vi "Teleop.vi"(10 "Match Info":T1={"Autonomous Elapsed Seconds"=0.0, "TeleOp Elapsed Seconds"=0.0, "Disabled Elapsed Seconds"=0.0, "Visited Autonomous"=FALSE, "Visited TeleOp"=FALSE, "Visited Disabled"=FALSE, "Autonomous Settings"={"Autonomous Style"=enum."Independent", "VI Refnum"=refnum}}, 11 "Call Context":T2) -> ()   [LabVIEW 2017]
doc: "This VI is called for each TeleOp packet received from the DS where the robot is not disabled. It is often used to read from the joysticks and update I/O or to update setpoints for timed control loops. It should complete and return within 20 milliseconds or it may miss DS packets."
uses:
  <vilib>/Rock Robotics/WPI/DriverStation/WPI_DriverStationDerivedRobotMode.ctl
  <vilib>/Rock Robotics/WPI/DriverStation/WPI_DriverStationMatch Info.ctl
  <vilib>/Rock Robotics/WPI/Utilities/WPI_GetSetVariantRefNum.vi
  <vilib>/Rock Robotics/Network Tables/NT Write Boolean Array.vi
  <vilib>/Rock Robotics/Network Tables/NT Write Numeric Array.vi
  <vilib>/Rock Robotics/Network Tables/NT Read Boolean.vi
  <vilib>/Rock Robotics/Network Tables/NT Read Number.vi
  Robot Global Data.vi
panel:
  out "Sample Slider 0":dbl(slide) scale=0.0..5.0
  out "Sample Boolean 1":bool
  out "Sample Boolean 0":bool
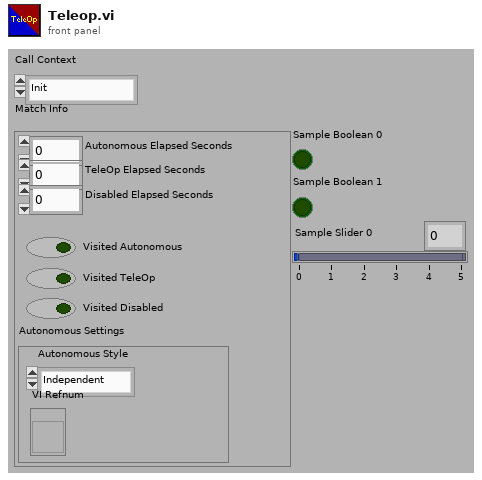
[diagram p1: front panel]
types:
  T1 = typedef "WPI_DriverStationMatch Info.ctl" = cluster{"Autonomous Elapsed Seconds":dbl, "TeleOp Elapsed Seconds":dbl, "Disabled Elapsed Seconds":dbl, "Visited Autonomous":bool, "Visited TeleOp":bool, "Visited Disabled":bool, "Autonomous Settings":cluster{"Autonomous Style":enum16{"Iterative", "Independent"}, "VI Refnum":refnum<vi>}}
  T2 = typedef "WPI_DriverStationDerivedRobotMode.ctl" = enum16{"Init", "Execute", "Stop"}
  T3 = typedef "WPI_JoystickDevRef.ctl" = cluster{"Device":T4}
  T4 = typedef "WPI_JoystickDeviceEnum.ctl" = enum16{"USB 0", "USB 1", "USB 2", "USB 3", "USB 4", "USB 5"}
  T5 = enum16{"SingleJoystick", "DoubleJoystick", "GameController"}
  T6 = cluster{"Buttons[0]":bool, "Buttons[1]":bool, "Buttons[2]":bool, "Buttons[3]":bool, "Buttons[4]":bool, "Buttons[5]":bool, "Buttons[6]":bool, "Buttons[7]":bool, "Buttons[8]":bool}
  T7 = cluster{"Axes[0]":dbl, "Axes[1]":dbl, "Axes[2]":dbl, "Axes[3]":dbl, "Axes[4]":dbl, "Axes[5]":dbl, "Axes[6]":dbl, "Axes[7]":dbl, "Axes[8]":dbl}
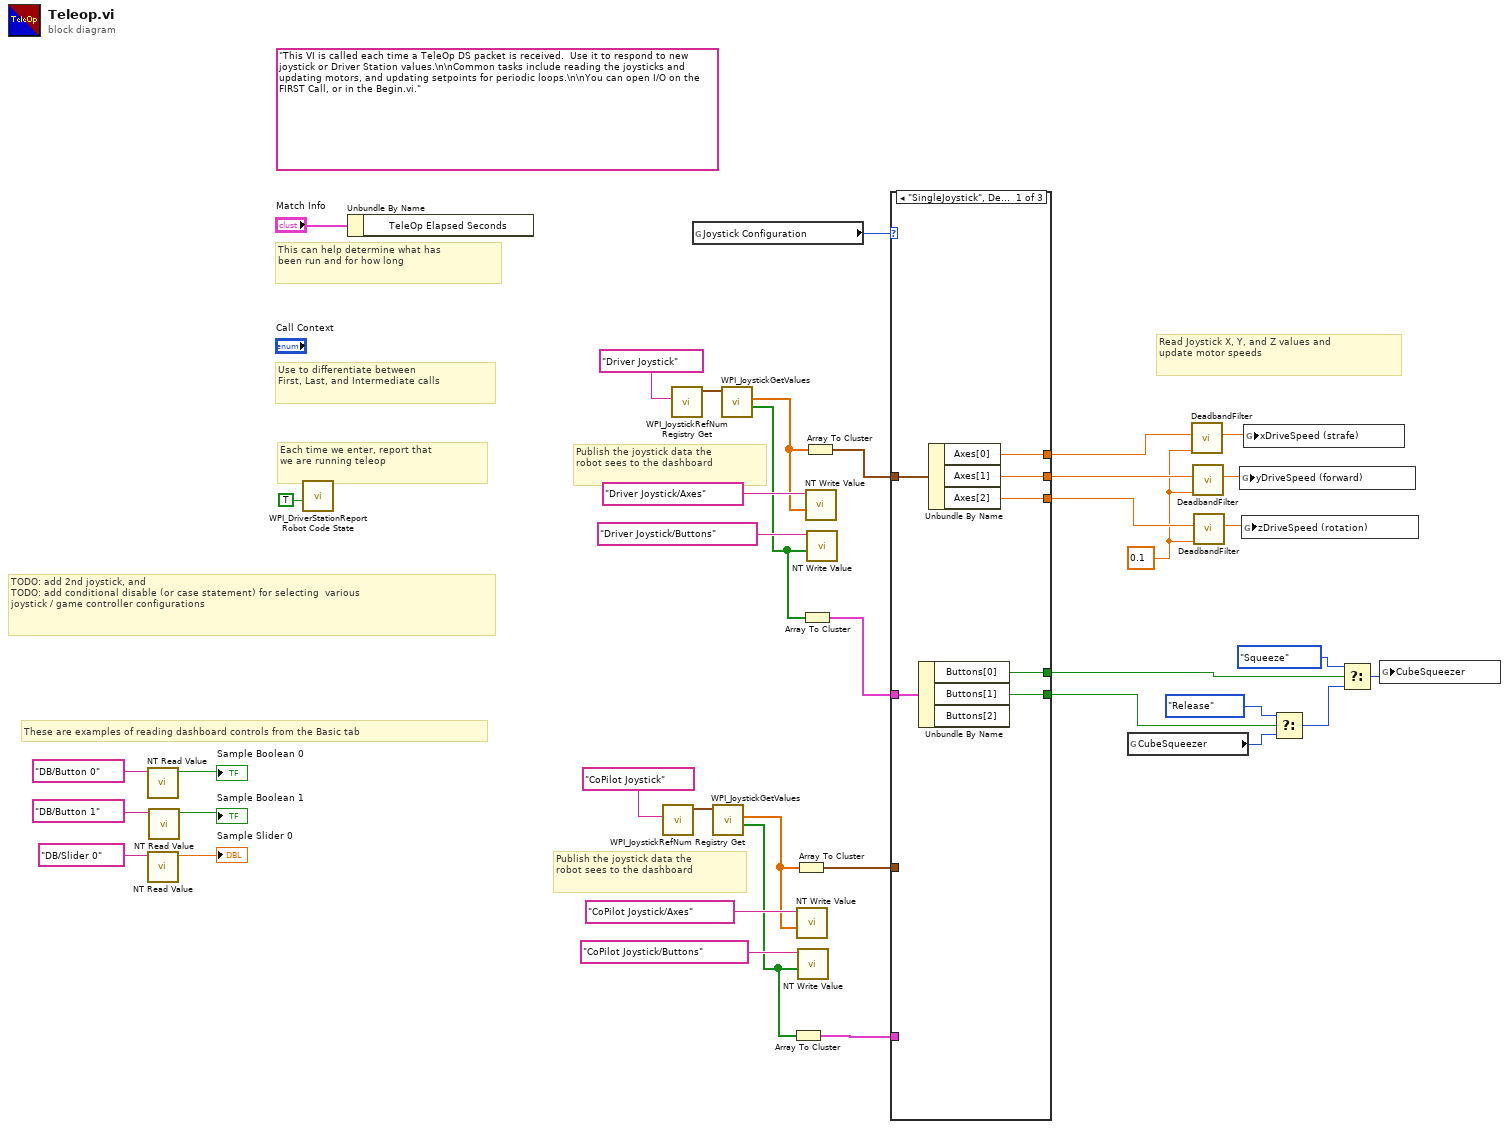
[diagram p0: block diagram]
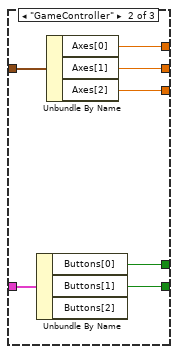
[diagram p2: hidden frame]
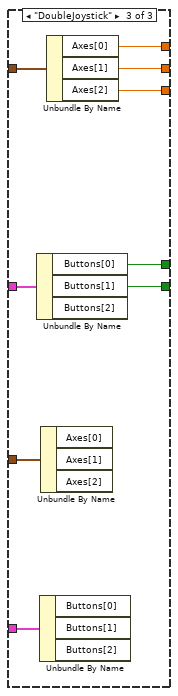
[diagram p3: hidden frame]
diagram:
  w15 = 0.1 ("guardband value")
  (unwired) "This VI is called each time a TeleOp DS packet is received.  Use it to respond to new joystick or Driver Station values.\n\nCommon tasks include reading the joysticks and updating motors, and updating setpoints for periodic loops.\n\nYou can open I/O on the FIRST Call, or in the Begin.vi."
  # "Publish the joystick data the\nrobot sees to the dashboard"
  # "TODO: add 2nd joystick, and \nTODO: add conditional disable (or case statement) for selecting  various \njoystick / game controller configurations"
  # "These are examples of reading dashboard controls from the Basic tab"
  # "Publish the joystick data the\nrobot sees to the dashboard"
  # "Each time we enter, report that\nwe are running teleop"
  # "Use to differentiate between\nFirst, Last, and Intermediate calls"
  # "This can help determine what has\nbeen run and for how long"
  # "Read Joystick X, Y, and Z values and \nupdate motor speeds"
  n1 = call-poly <vilib>:"NT Read Value.vi"("Name"="DB/Button 0" ("refnum name")) -> ("Boolean"=→"Sample Boolean 0":bool)  [unwired: 9 in, 1 out]
  n2 = call-poly <vilib>:"NT Read Value.vi"("Name"="DB/Slider 0" ("refnum name")) -> ("Numeric"=→"Sample Slider 0":dbl)  [unwired: 9 in, 1 out]
  n3 = call-poly <vilib>:"NT Read Value.vi"("Name"="DB/Button 1" ("refnum name")) -> ("Boolean"=→"Sample Boolean 1":bool)  [unwired: 9 in, 1 out]
  n4 = call <vilib>:"WPI_DriverStationReport Robot Code State.vi"("TeleOp"=TRUE ("Autonomous")) -> ()  [unwired: 10 in, 1 out]
  n5 = Unbundle By Name("Match Info") -> ()  [unwired: 1 out]
  n6 = call <vilib>:"WPI_JoystickRefNum Registry Get.vi"("refnum name"="CoPilot Joystick") -> ("JoystickDevRef"=w8:T3)  [unwired: 1 in, 9 out]
  n7 = call <vilib>:"WPI_JoystickRefNum Registry Get.vi"("refnum name"="Driver Joystick") -> ("JoystickDevRef"=w37:T3)  [unwired: 1 in, 9 out]
  n8 = global read "Robot Global Data.vi" "Joystick Configuration"() -> (w1:T5)
  n9 = call <vilib>:"WPI_JoystickGetValues.vi"("JoystickDevRef"=w8) -> ("Buttons"=w3:bool[], "Axes"=w5:dbl[])  [unwired: 6 in, 3 out]
  n10 = call <vilib>:"WPI_JoystickGetValues.vi"("JoystickDevRef"=w37) -> ("Buttons"=w25:bool[], "Axes"=w27:dbl[])  [unwired: 6 in, 3 out]
  n11 = Array To Cluster(array=w3) -> (cluster=w2:T6)
  n12 = Array To Cluster(array=w5) -> (cluster=w4:T7)
  n13 = call-poly <vilib>:"NT Write Value.vi"("Numeric Array"=w5, "Name"="CoPilot Joystick/Axes") -> ()  [unwired: 9 in, 1 out]
  n14 = call-poly <vilib>:"NT Write Value.vi"("Boolean Array"=w3, "Name"="CoPilot Joystick/Buttons") -> ()  [unwired: 9 in, 1 out]
  n15 = Array To Cluster(array=w25) -> (cluster=w24:T6)
  n16 = Array To Cluster(array=w27) -> (cluster=w26:T7)
  n17 = call-poly <vilib>:"NT Write Value.vi"("Numeric Array"=w27, "Name"="Driver Joystick/Axes") -> ()  [unwired: 9 in, 1 out]
  n18 = call-poly <vilib>:"NT Write Value.vi"("Boolean Array"=w25, "Name"="Driver Joystick/Buttons") -> ()  [unwired: 9 in, 1 out]
  n19 = case shown="\"SingleJoystick\", Default" w1 {
    tunnel: w26 -> [w46 w53 w62]
    tunnel: w24 -> [w45 w52 w61]
    tunnel: [w44 w51 w60] -> w20
    tunnel: [w43 w50 w59] -> w19
    tunnel: [w42 w49 w58] -> w18
    tunnel: [w41 w48 w57] -> w17
    tunnel: [w40 w47 w56] -> w16
    tunnel: w4 -> [_ _ w55]
    tunnel: w2 -> [_ _ w54]
    frame "SingleJoystick", Default {
      n20 = Unbundle By Name(w45) -> ("Buttons[0]"=w41:bool, "Buttons[1]"=w40:bool)  [unwired: 1 out]
      n21 = Unbundle By Name(w46) -> ("Axes[0]"=w44:dbl, "Axes[1]"=w43:dbl, "Axes[2]"=w42:dbl)
    }
    frame "GameController" {
      n22 = Unbundle By Name(w52) -> ("Buttons[0]"=w48:bool, "Buttons[1]"=w47:bool)  [unwired: 1 out]
      n23 = Unbundle By Name(w53) -> ("Axes[0]"=w51:dbl, "Axes[1]"=w50:dbl, "Axes[2]"=w49:dbl)
    }
    frame "DoubleJoystick" {
      n24 = Unbundle By Name(w61) -> ("Buttons[0]"=w57:bool, "Buttons[1]"=w56:bool)  [unwired: 1 out]
      n25 = Unbundle By Name(w54) -> ()  [unwired: 3 out]
      n26 = Unbundle By Name(w55) -> ()  [unwired: 3 out]
      n27 = Unbundle By Name(w62) -> ("Axes[0]"=w60:dbl, "Axes[1]"=w59:dbl, "Axes[2]"=w58:dbl)
    }
  }
  n28 = global read "Robot Global Data.vi" "CubeSqueezer"() -> (w14:enum16{"Squeeze", "Release"})
  n29 = call "DeadbandFilter.vi"("guardband value"=w15, "JoystickAxis"=w20) -> ("FilteredJoystickAxis"=w23:dbl)  [unwired: 9 in]
  n30 = call "DeadbandFilter.vi"("guardband value"=w15, "JoystickAxis"=w19) -> ("FilteredJoystickAxis"=w22:dbl)  [unwired: 9 in]
  n31 = call "DeadbandFilter.vi"("guardband value"=w15, "JoystickAxis"=w18) -> ("FilteredJoystickAxis"=w21:dbl)  [unwired: 9 in]
  n32 = global write "Robot Global Data.vi" "yDriveSpeed (forward)"(w22) -> ()
  n33 = global write "Robot Global Data.vi" "zDriveSpeed (rotation)"(w21) -> ()
  n34 = global write "Robot Global Data.vi" "xDriveSpeed (strafe)"(w23) -> ()
  n35 = Select(t=enum16{"Squeeze", "Release"}."Release" ("CubeSqueezer"), s=w16, f=w14) -> (s? t:f=w10:enum16{"Squeeze", "Release"})
  n36 = Select(t=enum16{"Squeeze", "Release"}."Squeeze" ("CubeSqueezer"), s=w17, f=w10) -> (s? t:f=w11:enum16{"Squeeze", "Release"})
  n37 = global write "Robot Global Data.vi" "CubeSqueezer"(w11) -> ()
